vi "get_coords.vi"(8 "error in (no error)":errorcluster, 11 "Waypoint in":refnum<class "Waypoint.lvclass">) -> (0 "error out":errorcluster, 2 "Coords":cluster{"X":dbl, "Y":dbl}, 3 "Waypoint out":refnum<class "Waypoint.lvclass">)   [LabVIEW 2011, in "Waypoint.lvclass"]
uses:
  Waypoint.lvclass
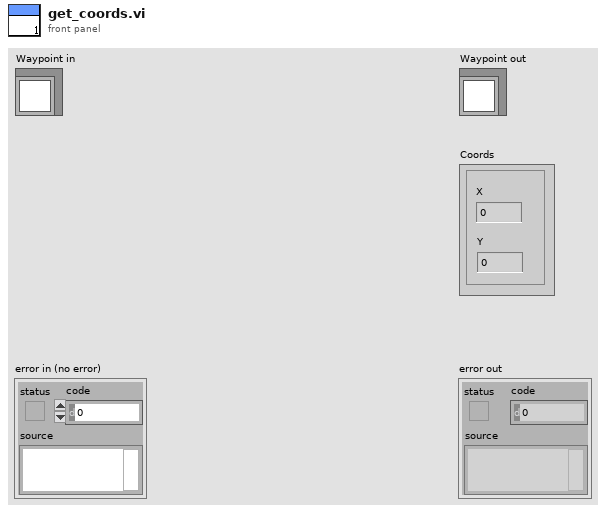
[diagram p1: front panel]
types:
  T1 = typedef "UTM Location.ctl" = cluster{"UTM Zone":dbl, "Hemisphere":enum16{"North", "South"}, "East":dbl, "North":dbl}
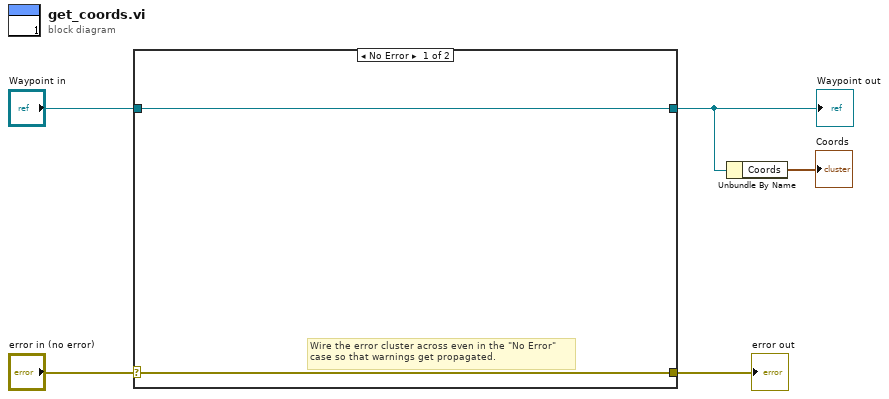
[diagram p0: block diagram]
diagram:
  n1 = case shown="No Error" "error in (no error)" {
    selector: "error in (no error)" -> [w7 w9]
    tunnel: [w7 w9] -> w4
    tunnel: [w6 w8] -> w2
    tunnel: "Waypoint in" -> [w6 w8]
    frame No Error {
      # "Wire the error cluster across even in the \"No Error\"\ncase so that warnings get propagated."
    }
    frame Error {
    }
  }
  "error out" <- w4
  "Waypoint out" <- w2
  n2 = Unbundle By Name(w2) -> ("Coords"=→"Coords":T1)
